vi "FPGA_Incremental_Enc.vi"(9 "Position Reset":bool, 10 "Velocity Interval (uSec)":u32=1000, 11 "Loop Timer DAQ":u32=1 caption="Loop Time(uSec)") -> (3 "Position (Counts)":i64)   [LabVIEW 2019]
uses:
  Custom Controls/Encoder_Pins.ctl
  <vilib>/rvi/Emulation/niFpgaSctlEmulationGetInTimedLoop.vi
  <vilib>/rvi/Emulation/niFpgaProcessEmulError.vi
  <vilib>/rvi/Emulation/niFpgaGetClockAttributes.vi
  <vilib>/rvi/Emulation/niFpgaEmulationReportErrorSimple.vi
  <vilib>/rvi/eio/common/nirviEmuTemplateMethod_errors.vi
  <vilib>/rvi/Emulation/niFpgaCriticalErrorInLSC.vi
  <vilib>/eio/EIONode/EIONode.xnode
panel:
  out "ConnectorA/DIO9":bool
  out "ConnectorA/DIO8":bool
  out "ConnectorA/DIO10":bool
  out "ConnectorA/DIO11":bool
  out "ConnectorA/DIO13":bool
  out "ConnectorA/DIO12":bool
  out "ConnectorA/DIO15":bool
  out "ConnectorA/DIO14":bool
  in  "Encoder Pins":T1
  out "A'":bool
  out "B'":bool
  out "A":bool
  out "B":bool
  in  "stop":bool
  in  "Debug: ConnectorA/DIO14":bool
  in  "Debug: ConnectorA/DIO15":bool
  in  "Debug":bool
  out "ticks":i64
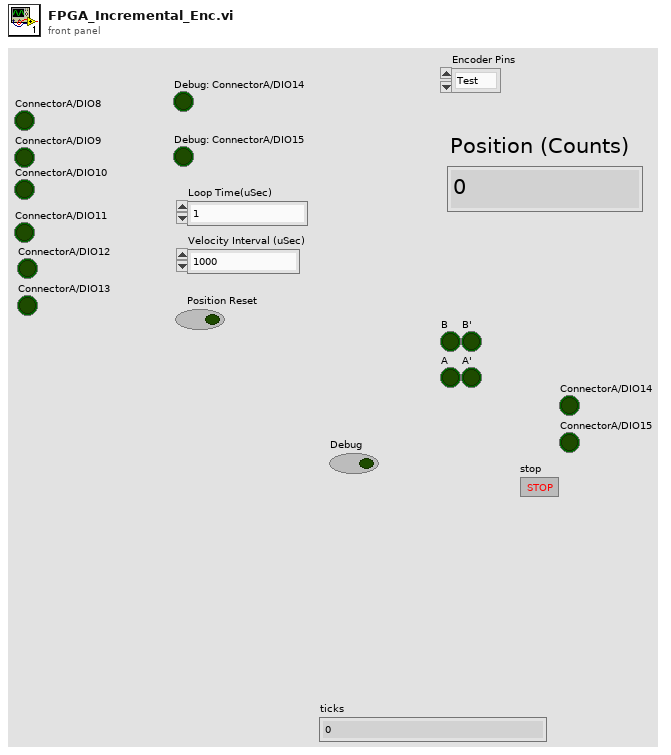
[diagram p1: front panel]
types:
  T1 = typedef "Encoder_Pins.ctl" = enum16{"Test", "Linear 1", "Linear 2", "Rotor 1", "Rotor 2"}
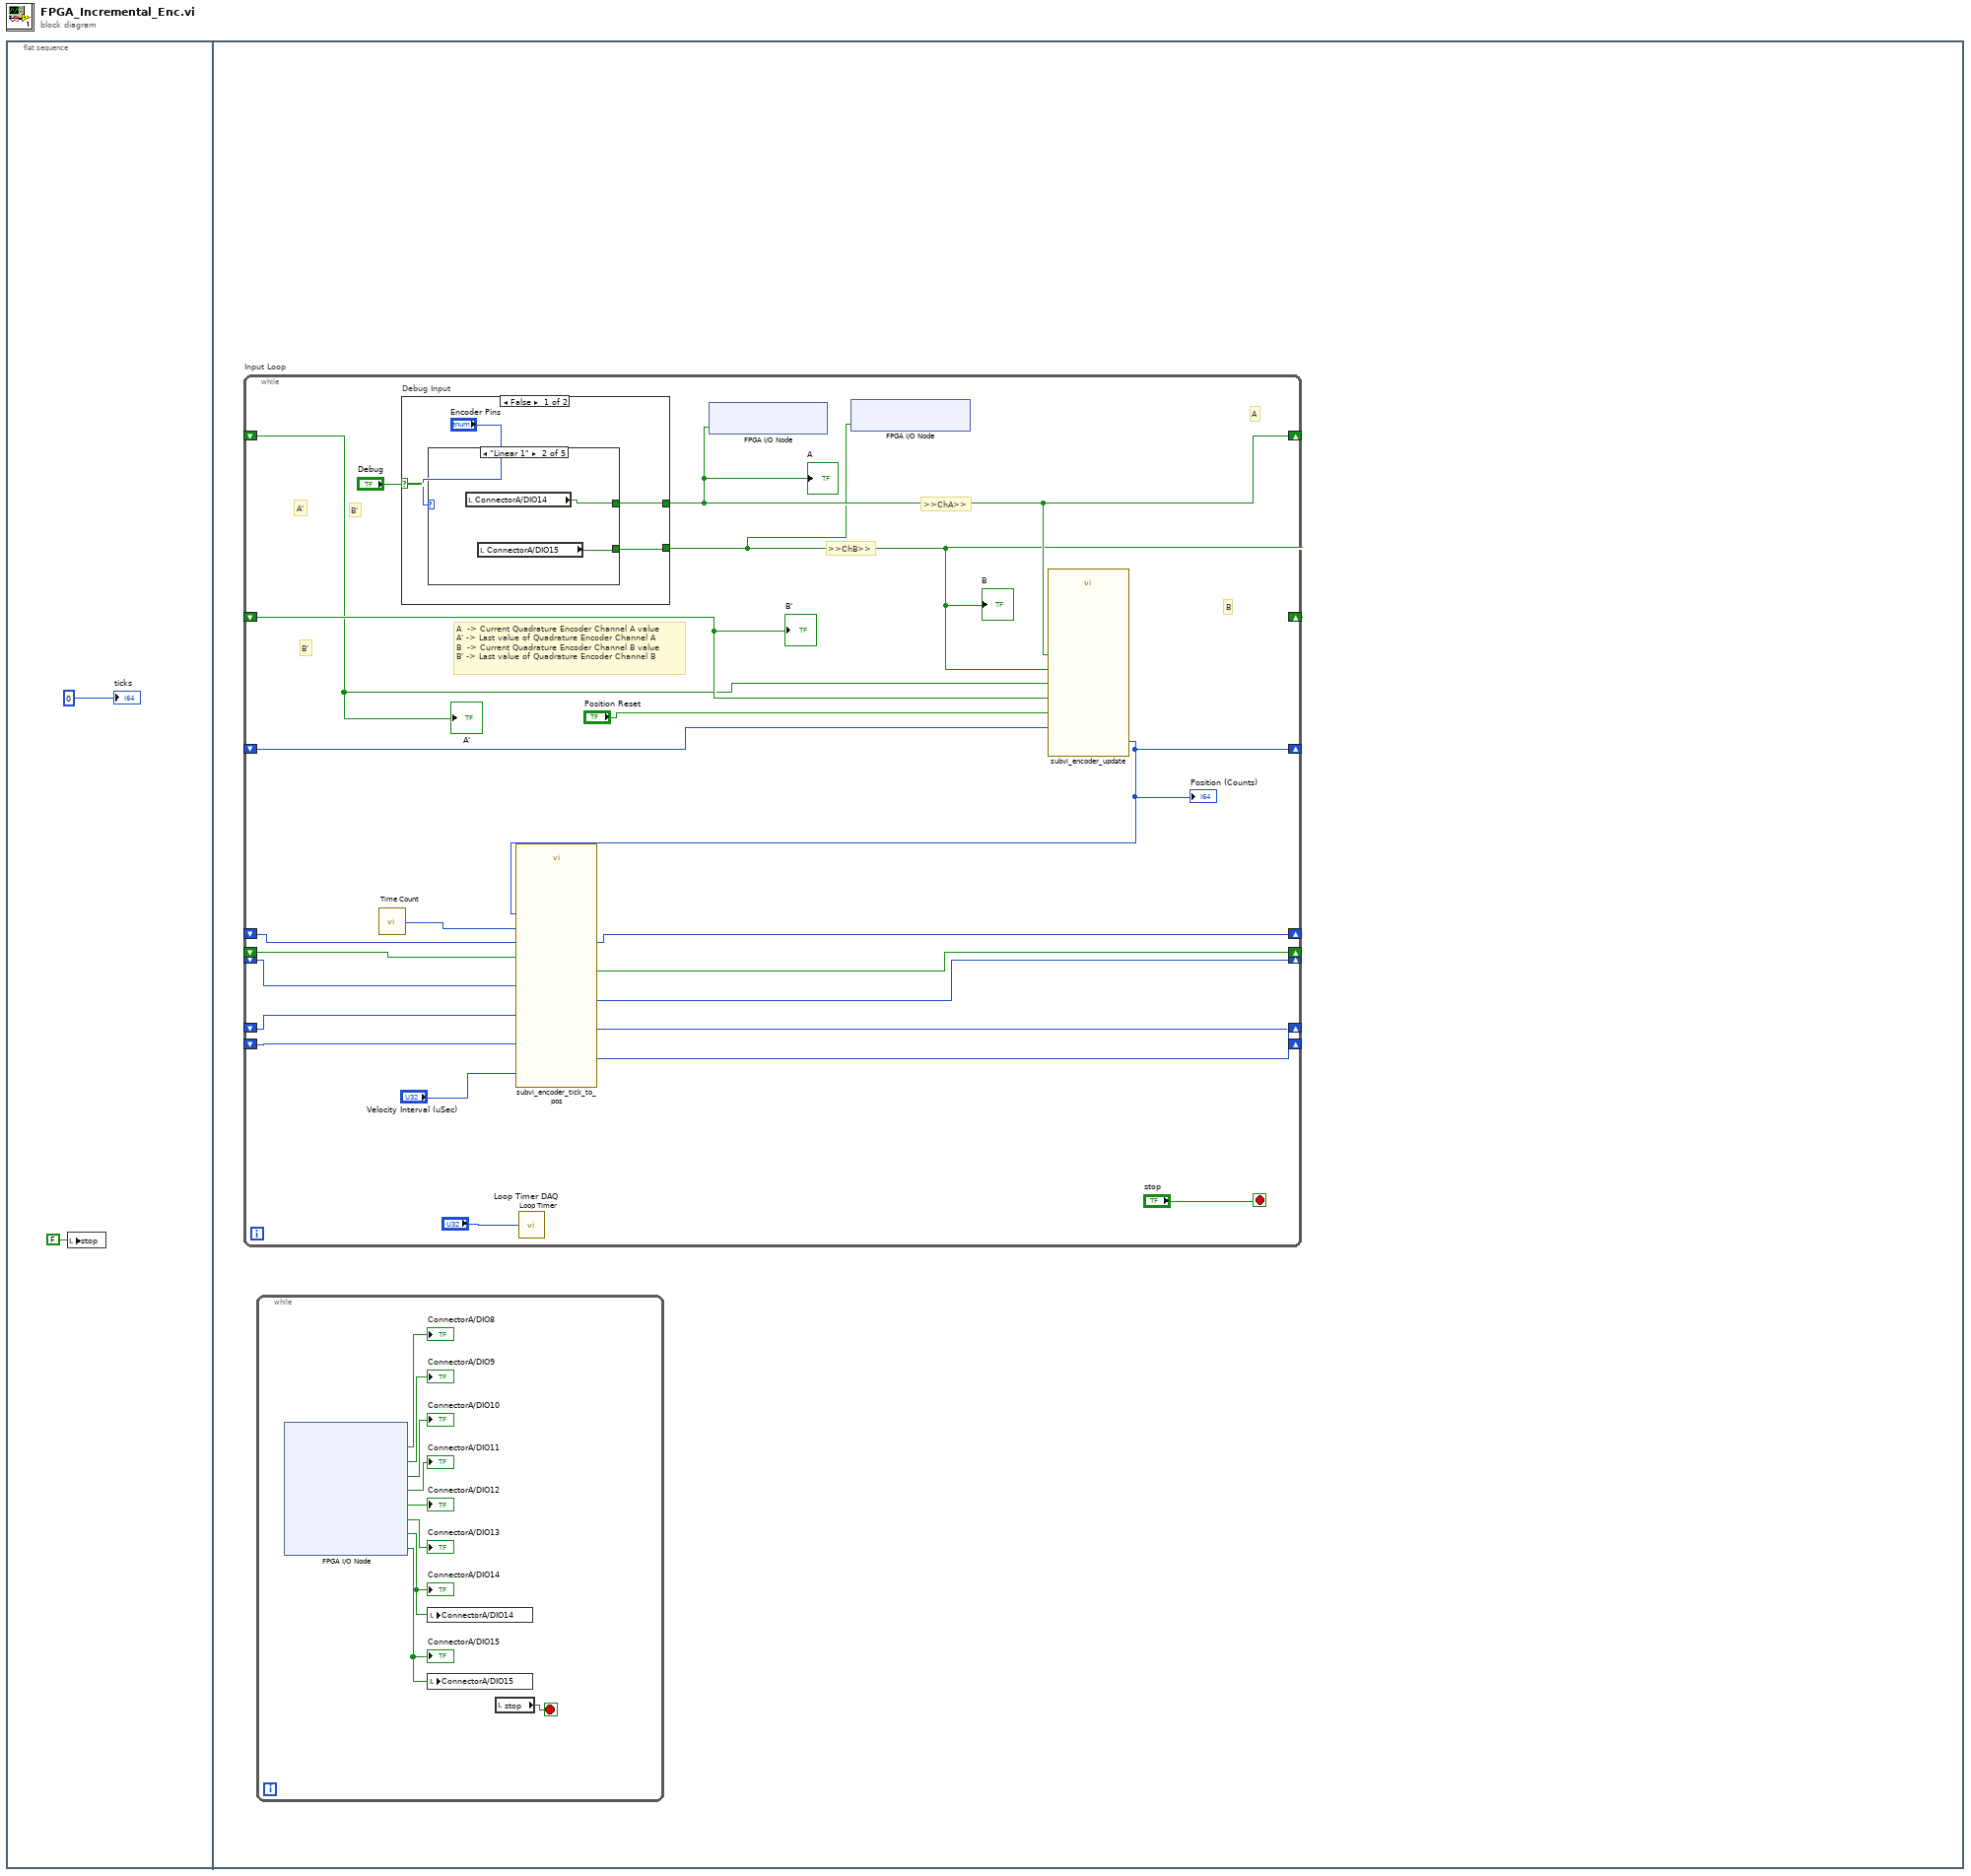
[diagram p0: block diagram]
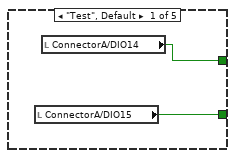
[diagram p2: hidden frame]
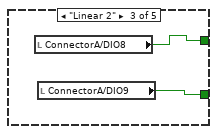
[diagram p3: hidden frame]
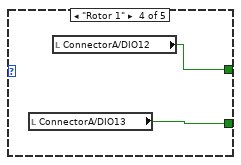
[diagram p4: hidden frame]
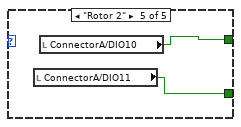
[diagram p5: hidden frame]
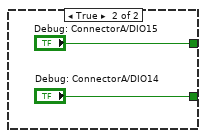
[diagram p6: hidden frame]
diagram:
  n1 = flat-sequence {
    frame #0 {
      n2 = local write "stop"(FALSE ("stop")) -> ()
      "ticks" <- i64 0 ("Numeric")
    }
    frame #1 {
      n3 = while "Input Loop" {
        shift-right: [w12] -> _
        shift-left: _ -> [w30]
        shift-right: [w13] -> _
        shift-left: _ -> [w29]
        shift-right: [w21] -> _
        shift-left: _ -> [w28]
        shift-right: [w26] -> _
        shift-left: _ -> [w25]
        shift-right: [w24] -> _
        shift-left: _ -> [w23]
        shift-right: [w22] -> _
        shift-left: _ -> [w20]
        shift-right: [w19] -> _
        shift-left: _ -> [w18]
        shift-right: [w17] -> _
        shift-left: _ -> [w16]
        stop <- "stop" stop-if-true
        # "B'"
        # ">>ChB>>"
        # ">>ChA>>"
        # "A'"
        # "A  -> Current Quadrature Encoder Channel A value\nA' -> Last value of Quadrature Encoder Channel A\nB  -> Current Quadrature Encoder Channel B value\nB' -> Last value of Quadrature Encoder Channel B"
        # "B'"
        # "B"
        # "A"
        n4 = call "Time Count"() -> ("Tick Count(uSec)"=w15:u32)
        n5 = case "Debug Input" shown="False" "Debug" {
          tunnel: [w35 "Debug: ConnectorA/DIO15"] -> w13
          tunnel: [w34 "Debug: ConnectorA/DIO14"] -> w12
          frame False {
            n6 = case shown="\"Linear 1\"" "Encoder Pins" {
              tunnel: [w38 w40 w42 w44 w46] -> w35
              tunnel: [w37 w39 w41 w43 w45] -> w34
              frame "Test", Default {
                n7 = local read "ConnectorA/DIO15"() -> (w37:bool)
                n8 = local read "ConnectorA/DIO14"() -> (w38:bool)
              }
              frame "Linear 1" {
                n9 = local read "ConnectorA/DIO14"() -> (w40:bool)
                n10 = local read "ConnectorA/DIO15"() -> (w39:bool)
              }
              frame "Linear 2" {
                n11 = local read "ConnectorA/DIO8"() -> (w42:bool)
                n12 = local read "ConnectorA/DIO9"() -> (w41:bool)
              }
              frame "Rotor 1" {
                n13 = local read "ConnectorA/DIO13"() -> (w43:bool)
                n14 = local read "ConnectorA/DIO12"() -> (w44:bool)
              }
              frame "Rotor 2" {
                n15 = local read "ConnectorA/DIO11"() -> (w45:bool)
                n16 = local read "ConnectorA/DIO10"() -> (w46:bool)
              }
            }
          }
          frame True {
          }
        }
        "B" <- w12
        "A" <- w13
        n17 = call "Loop Timer"("Count(uSec)"="Loop Timer DAQ") -> ()  [unwired: 1 out]
        n18 = xnode "FPGA I/O Node"("ConnectorA/DIO0"=w13) -> ()  [unwired: 1 in, 1 out]
        n19 = xnode "FPGA I/O Node"("ConnectorA/DIO1"=w12) -> ()  [unwired: 1 in, 1 out]
        n20 = call "subvi_encoder_update.vi"("Position Reset"="Position Reset", "Tick'"=w28, "A"=w13, "B'"=w30, "A'"=w29, "B"=w12) -> ("Tick"=w21:i32)  [unwired: 5 in]
        "Position (Counts)" <- w21
        n21 = call "subvi_encoder_tick_to_pos.vi"("Velocity Interval (uSec)"="Velocity Interval (uSec)", "Raw Tick"=w21, "Waited?'"=w18, "Tick Count(uSec)'"=w16, "p'"=w20, "Time Count"=w15, "a'"=w23, "v'"=w25) -> ("Waited?"=w19:bool, "Tick Count(uSec)"=w17:u32, "p"=w22:i32, "a"=w24:i32, "v"=w26:i32)  [unwired: 3 in]
        "B'" <- w30
        "A'" <- w29
      }
      n22 = while {
        stop <- w9 stop-if-true
        n23 = xnode "FPGA I/O Node"() -> ("ConnectorA/DIO8"=→"ConnectorA/DIO8":bool, "ConnectorA/DIO9"=→"ConnectorA/DIO9":bool, "ConnectorA/DIO10"=→"ConnectorA/DIO10":bool, "ConnectorA/DIO11"=→"ConnectorA/DIO11":bool, "ConnectorA/DIO12"=→"ConnectorA/DIO12":bool, "ConnectorA/DIO13"=→"ConnectorA/DIO13":bool, "ConnectorA/DIO14"=w10:bool, "ConnectorA/DIO15"=w11:bool)  [unwired: 8 in, 8 out]
        "ConnectorA/DIO14" <- w10
        "ConnectorA/DIO15" <- w11
        n24 = local write "ConnectorA/DIO14"(w10) -> ()
        n25 = local write "ConnectorA/DIO15"(w11) -> ()
        n26 = local read "stop"() -> (w9:bool)
      }
    }
  }
